vi "gfitsio-check-image-for-read.vi"(4 "lpixel":i32[](array[numeric]), 5 "inc":i32[](array[numeric]), 6 "fpixel":i32[](array[numeric]), 8 "error in (no error)":errorcluster, 11 "gfits refnum":T1) -> (0 "error out":errorcluster, 1 "lpixel out":i32[](array[numeric]), 3 "dup gfits refnum":T1)   [LabVIEW 2011, in "gfitsio.lvlib"]
uses:
  gfitsio.lvlib
  gfitsio-refnum.ctl
panel:
  # "If -1 is supplied for lpixel this VI returns the actual lpixel of the image."
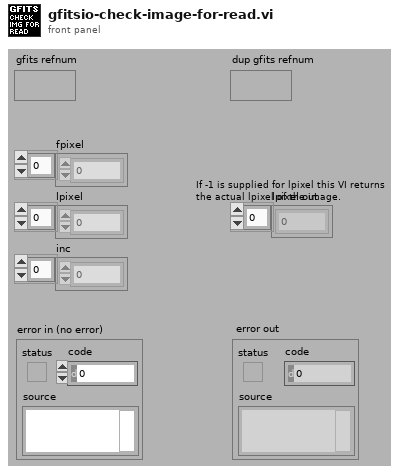
[diagram p1: front panel]
types:
  T1 = typedef "gfitsio.lvlib/gfitsio-refnum.ctl" = refnum<k1>
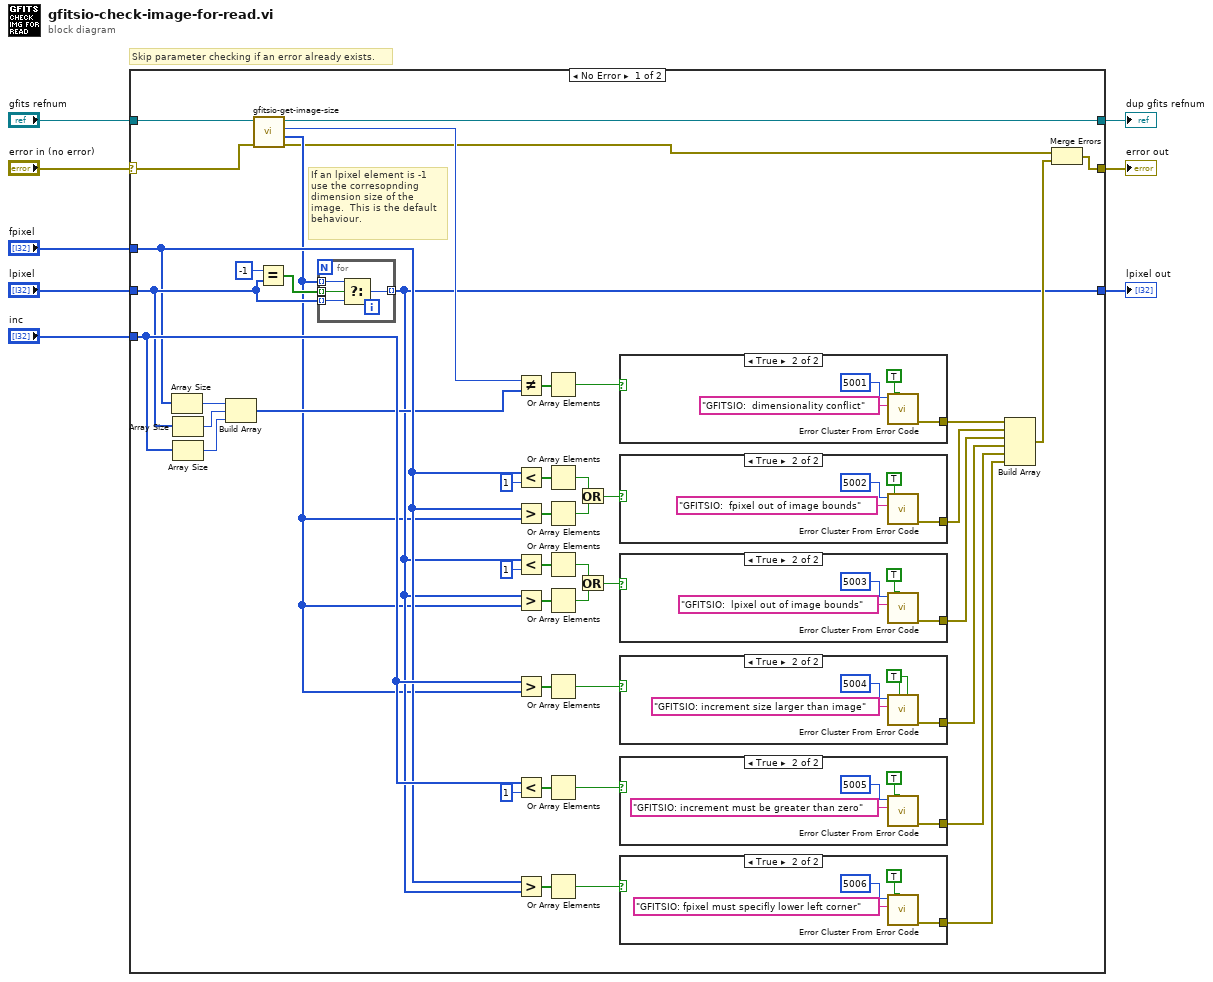
[diagram p0: block diagram]
diagram:
  # "Skip parameter checking if an error already exists."
  n1 = case shown="No Error" "error in (no error)" {
    selector: "error in (no error)" -> [w52 w84]
    tunnel: "gfits refnum" -> [w53 w83]
    tunnel: [w9 w83] -> w3
    tunnel: "fpixel" -> [w19 _]
    tunnel: "lpixel" -> [w20 w82]
    tunnel: "inc" -> [w21 _]
    tunnel: [w51 w84] -> w8
    tunnel: [w12 w82] -> w1
    frame No Error {
      # "If an lpixel element is -1 use the corresopnding dimension size of the image.  This is the default behaviour."
      n2 = Array Size(array=w19) -> (size(s)=w18:i32)
      n3 = Array Size(array=w20) -> (size(s)=w17:i32)
      n4 = Array Size(array=w21) -> (size(s)=w16:i32)
      n5 = Build Array(w18, w17, w16) -> (w15:i32[])
      n6 = call "gfitsio-get-image-size.vi"("error in (no error)"=w52, "gfits refnum"=w53) -> ("error out"=w10:errorcluster, "naxes"=w11:i32[], "naxis"=w48:i32, "dup gfits refnum"=w9:T1)  [unwired: 6 in]
      n7 = Equal?(x=-1, y=w20) -> (x = y?=w22:bool[])
      n8 = for {
        tunnel: w11 -> [w56] mode=indexing
        tunnel: w22 -> [w55] mode=indexing
        tunnel: w20 -> [w57] mode=indexing
        tunnel: [w54] -> w12 mode=indexing
        n9 = Select(t=w56, s=w55, f=w57) -> (s? t:f=w54:i32)
      }
      n10 = Not Equal?(x=w48, y=w15) -> (x != y?=w14:bool[])
      n11 = Less?(x=w19, y=1 ("x")) -> (x < y?=w42:bool[])
      n12 = Greater?(x=w19, y=w11) -> (0:w41:bool[])
      n13 = Less?(x=w12, y=1 ("x")) -> (x < y?=w34:bool[])
      n14 = Greater?(x=w12, y=w11) -> (0:w35:bool[])
      n15 = Greater?(x=w21, y=w11) -> (0:w27:bool[])
      n16 = Less?(x=w21, y=1 ("x")) -> (x < y?=w29:bool[])
      n17 = Greater?(x=w19, y=w12) -> (0:w25:bool[])
      n18 = Or Array Elements(Boolean array=w14) -> (logical OR=w13:bool)
      n19 = Or Array Elements(Boolean array=w42) -> (logical OR=w39:bool)
      n20 = Or Array Elements(Boolean array=w41) -> (logical OR=w38:bool)
      n21 = Or Array Elements(Boolean array=w34) -> (logical OR=w36:bool)
      n22 = Or Array Elements(Boolean array=w35) -> (logical OR=w37:bool)
      n23 = Or Array Elements(Boolean array=w27) -> (logical OR=w26:bool)
      n24 = Or Array Elements(Boolean array=w29) -> (logical OR=w28:bool)
      n25 = Or Array Elements(Boolean array=w25) -> (logical OR=w24:bool)
      n26 = Or(x=w39, y=w38) -> (x .or. y?=w40:bool)
      n27 = Or(x=w36, y=w37) -> (x .or. y?=w32:bool)
      n28 = case shown="True" w13 {
        tunnel: [_ w79] -> w50
        frame False {
        }
        frame True {
          n29 = call <vilib>:"Error Cluster From Error Code.vi"("show call chain? (False)"=TRUE, "error message (\"\")"="GFITSIO:  dimensionality conflict" ("error message (\"\")"), "error code (0)"=5001) -> ("error out"=w79:errorcluster)  [unwired: 6 in]
        }
      }
      n30 = case shown="True" w40 {
        tunnel: [_ w75] -> w47
        frame False {
        }
        frame True {
          n31 = call <vilib>:"Error Cluster From Error Code.vi"("show call chain? (False)"=TRUE, "error message (\"\")"="GFITSIO:  fpixel out of image bounds" ("error message (\"\")"), "error code (0)"=5002) -> ("error out"=w75:errorcluster)  [unwired: 6 in]
        }
      }
      n32 = case shown="True" w32 {
        tunnel: [_ w71] -> w46
        frame False {
        }
        frame True {
          n33 = call <vilib>:"Error Cluster From Error Code.vi"("show call chain? (False)"=TRUE, "error message (\"\")"="GFITSIO:  lpixel out of image bounds" ("error message (\"\")"), "error code (0)"=5003) -> ("error out"=w71:errorcluster)  [unwired: 6 in]
        }
      }
      n34 = case shown="True" w26 {
        tunnel: [_ w67] -> w45
        frame False {
        }
        frame True {
          w66 = TRUE ("show call chain? (False)")
          n35 = call <vilib>:"Error Cluster From Error Code.vi"("is warning? (False)"=w66, "show call chain? (False)"=w66, "error message (\"\")"="GFITSIO: increment size larger than image" ("error message (\"\")"), "error code (0)"=5004) -> ("error out"=w67:errorcluster)  [unwired: 5 in]
        }
      }
      n36 = case shown="True" w28 {
        tunnel: [_ w63] -> w44
        frame False {
        }
        frame True {
          n37 = call <vilib>:"Error Cluster From Error Code.vi"("show call chain? (False)"=TRUE, "error message (\"\")"="GFITSIO: increment must be greater than zero" ("error message (\"\")"), "error code (0)"=5005) -> ("error out"=w63:errorcluster)  [unwired: 6 in]
        }
      }
      n38 = case shown="True" w24 {
        tunnel: [_ w59] -> w31
        frame False {
        }
        frame True {
          n39 = call <vilib>:"Error Cluster From Error Code.vi"("show call chain? (False)"=TRUE, "error message (\"\")"="GFITSIO: fpixel must specifly lower left corner" ("error message (\"\")"), "error code (0)"=5006) -> ("error out"=w59:errorcluster)  [unwired: 6 in]
        }
      }
      n40 = Build Array(w50, w47, w46, w45, w44, w31) -> (w49:errorcluster[])
      n41 = Merge Errors(w10, w49) -> (w51:errorcluster)
    }
    frame Error {
    }
  }
  "error out" <- w8
  "dup gfits refnum" <- w3
  "lpixel out" <- w1
